vi "AIT 664 - RT Driver Init.vi"(0 "Device Reference in":T1 format="%.0x", 11 "error in":errorcluster) -> (4 "Device Reference out":T1 format="%.0x", 6 "End System Handle out":u64 format="%x", 15 "error out":errorcluster)   [LabVIEW 2014, in "AIT 664 Custom Device.lvlib"]
doc: "Configure AIT 664 card via VISA address, load .HEX configuration file, and set AIT 664 dateTime.\n\nReturns handle to AIT 664 card.\n\nError - error 5555 if VISA address is not set."
uses:
  AIT 664 Custom Device.lvlib
  <vilib>/NI Veristand/Custom Device API/Custom Device Item Ref.ctl
  <instrlib>/AIT 664/Private/AIT 664 Configure/AIT 664 Configure End System (1HEX).vi
  <instrlib>/AIT 664/Private/AIT 664 Initialize/AIT 664 Initialize (VISADeviceName).vi
  <vilib>/NI Veristand/Custom Device API/Get Item Property (String).vi
  Controls and Global/Global.vi
  <vilib>/NI Veristand/Custom Device API/Custom Device API.lvlib
  <instrlib>/AIT 664/AIT 664.lvlib
  <vilib>/NI Veristand/Custom Device Tools/Custom Device Utility Library/Custom Device Utility Library.lvlib
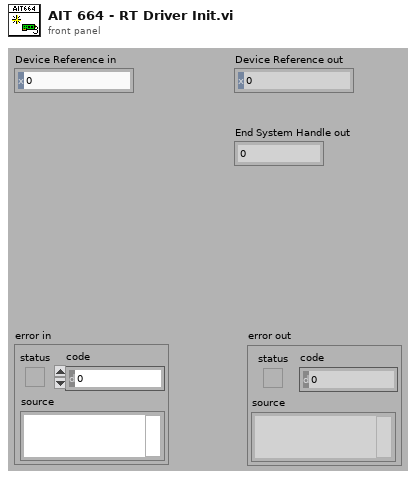
[diagram p1: front panel]
types:
  T1 = typedef "Custom Device API.lvlib/Custom Device Item Ref.ctl" = u64
  T2 = cluster{"Day":u32, "Hour":u32, "Min.":u32, "Sec.":u32, "Nanosecond":u32}
  T3 = typedef "LVDateTimeRec.ctl" = cluster{"fractional second":dbl, "second":i32, "minute":i32, "hour":i32, "day of month":i32, "month":i32, "year":i32, "day of week":i32, "day of year":i32, "DST":i32}
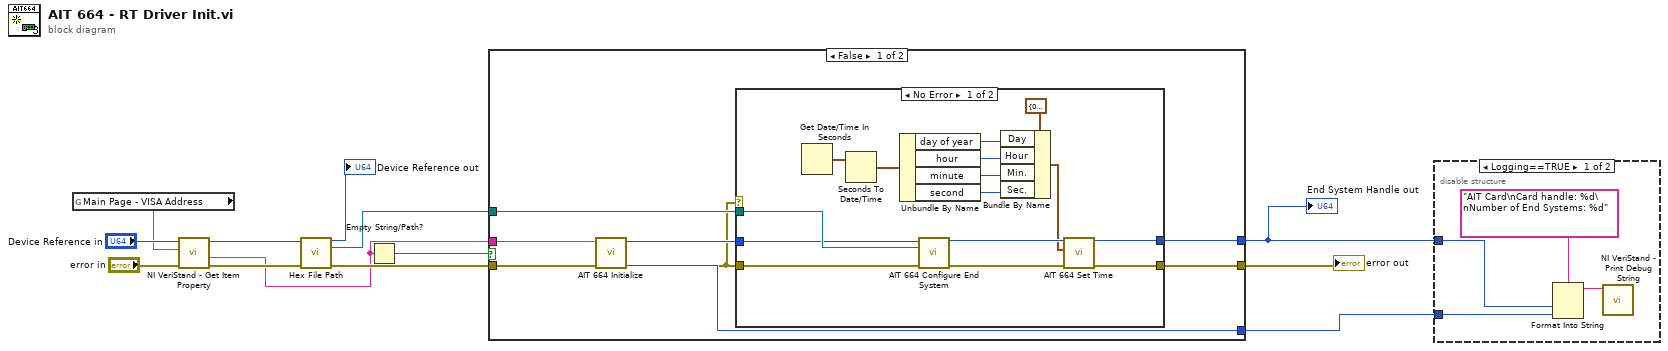
[diagram p0: block diagram]
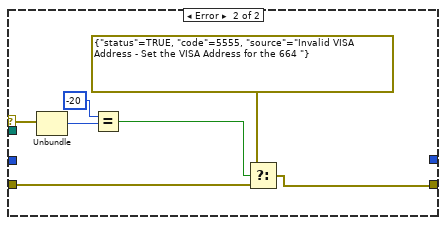
[diagram p3: hidden frame]
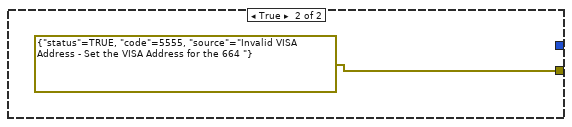
[diagram p4: hidden frame]
diagram:
  n1 = global read "Global.vi" "Main Page - VISA Address"() -> (w4:string)
  n2 = call-poly <vilib>:"NI VeriStand - Get Item Property.vi"("error in (no error)"="error in", "Property Name"=w4, "Item Ref in"="Device Reference in") -> ("error out"=w13:errorcluster, "Value"=w3:string, "Item Ref out"=w12:T1)  [unwired: 5 in, 1 out]
  n3 = call "Hex File Path.vi"("Device Reference in"=w12, "error in (no error)"=w13) -> ("Device Reference out"=→"Device Reference out":T1, "appended path"=w8:path, "error out"=w7:errorcluster)  [unwired: 11 in]
  n4 = Empty String/Path?(string/path=w3) -> (empty?=w2:bool)
  n5 = case shown="False" w2 {
    tunnel: w8 -> [w21 _]
    tunnel: w7 -> [w20 _]
    tunnel: [w19 _] -> w6
    tunnel: [w16 _] -> w5
    tunnel: [w17 errorcluster {"status"=TRUE, "code"=5555, "source"="Invalid VISA Address - Set the VISA Address for the 664 "} ("error out")] -> w1
    tunnel: w3 -> [w18 _]
    frame False {
      n6 = call-poly <instrlib>:"AIT 664 Initialize.vi"("VISA Device Name"=w18, "error in"=w20) -> ("End System Handle out"=w15:u64, "Number End Systems out"=w19:u32, "error out"=w14:errorcluster)  [unwired: 6 in]
      n7 = case shown="No Error" w14 {
        selector: w14 -> [_ w43]
        tunnel: w21 -> [w36 _]
        tunnel: w14 -> [w35 w38]
        tunnel: [w34 w37] -> w17
        tunnel: [w32 _] -> w16
        tunnel: w15 -> [w23 _]
        frame No Error {
          n8 = Get Date/Time In Seconds() -> (seconds since 1Jan1904=w26:timestamp)
          n9 = Seconds To Date/Time(time stamp (now)=w26) -> (date time rec=w25:T3)  [unwired: 1 in]
          n10 = Unbundle By Name(w25) -> ("day of year"=w28:i32, "hour"=w29:i32, "minute"=w30:i32, "second"=w31:i32)
          n11 = call-poly <instrlib>:"AIT 664 Configure End System.vi"("End System Handle in"=w23, "End System HEX Configuration File in"=w36, "error in"=w35) -> ("End System Handle out"=w33:u64, "error out"=w22:errorcluster)  [unwired: 11 in]
          n12 = Bundle By Name(cluster=T2 {"Day"=0, "Hour"=0, "Min."=0, "Sec."=0, "Nanosecond"=0} ("Time"), "Day"=w28, "Hour"=w29, "Min."=w30, "Sec."=w31) -> (w24:T2)
          n13 = call <instrlib>:"AIT 664 Set Time.vi"("error in"=w22, "Time"=w24, "End System Handle in"=w33) -> ("error out"=w34:errorcluster, "End System Handle out"=w32:u64)  [unwired: 7 in]
        }
        frame Error {
          n14 = Unbundle(w43) -> ("code"=w42:i32)  [unwired: 2 out]
          n15 = Equal?(x=-20, y=w42) -> (x = y?=w40:bool)
          n16 = Select(t=errorcluster {"status"=TRUE, "code"=5555, "source"="Invalid VISA Address - Set the VISA Address for the 664 "} ("error out"), s=w40, f=w38) -> (s? t:f=w37:errorcluster)
        }
      }
    }
    frame True {
    }
  }
  "error out" <- w1
  "End System Handle out" <- w5
  n17 = disable-structure shown="Logging==TRUE" {
    disable-tunnel: w6 -> [w47 _]
    disable-tunnel: w5 -> [w46 _]
    frame condition #0 (active) {
      n18 = Format Into String(format string="AIT Card\nCard handle: %d\nNumber of End Systems: %d", w46, w47) -> (resulting string=w45:string)  [unwired: 2 in, 1 out]
      n19 = call <vilib>:"NI VeriStand - Print Debug String.vi"("Message"=w45) -> ()  [unwired: 10 in, 1 out]
    }
    frame condition #1 {
    }
  }
